vi "FirstCall.vi"(9 "input":dbl) -> (1 "output":dbl, 3 "初始化":string)   [LabVIEW 2011]
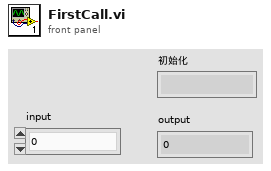
[diagram p1: front panel]
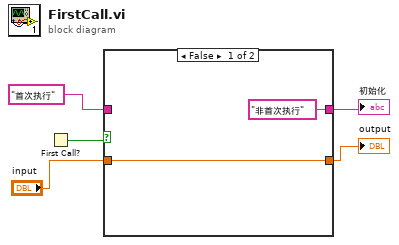
[diagram p0: block diagram]
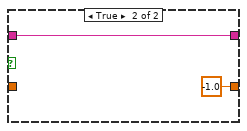
[diagram p2: hidden frame]
diagram:
  n1 = First Call?() -> (First Call?: T/F=w5:bool)
  n2 = case shown="False" w5 {
    tunnel: "首次执行" -> [_ w8]
    tunnel: [w7 -1.0 ("input")] -> w3
    tunnel: "input" -> [w7 _]
    tunnel: ["非首次执行" w8] -> w1
    frame False {
    }
    frame True {
    }
  }
  "output" <- w3
  "初始化" <- w1
